vi "VI Tree.vi"   [LabVIEW 2016, in "Error Manager.lvlib"]
doc: "VI Tree\nThis VI lists all the public VIs and CTLs of the library."
uses:
  Error Manager.lvlib
  Show Error Window Instruction (enum).ctl
panel:
  # "VI Tree\nSee the block diagram for the VI Tree"
types:
  T1 = typedef "Error Manager.lvlib/Show Error Window Instruction (enum).ctl" = enum16{"Use Default Setting", "Show", "Do Not Show"}
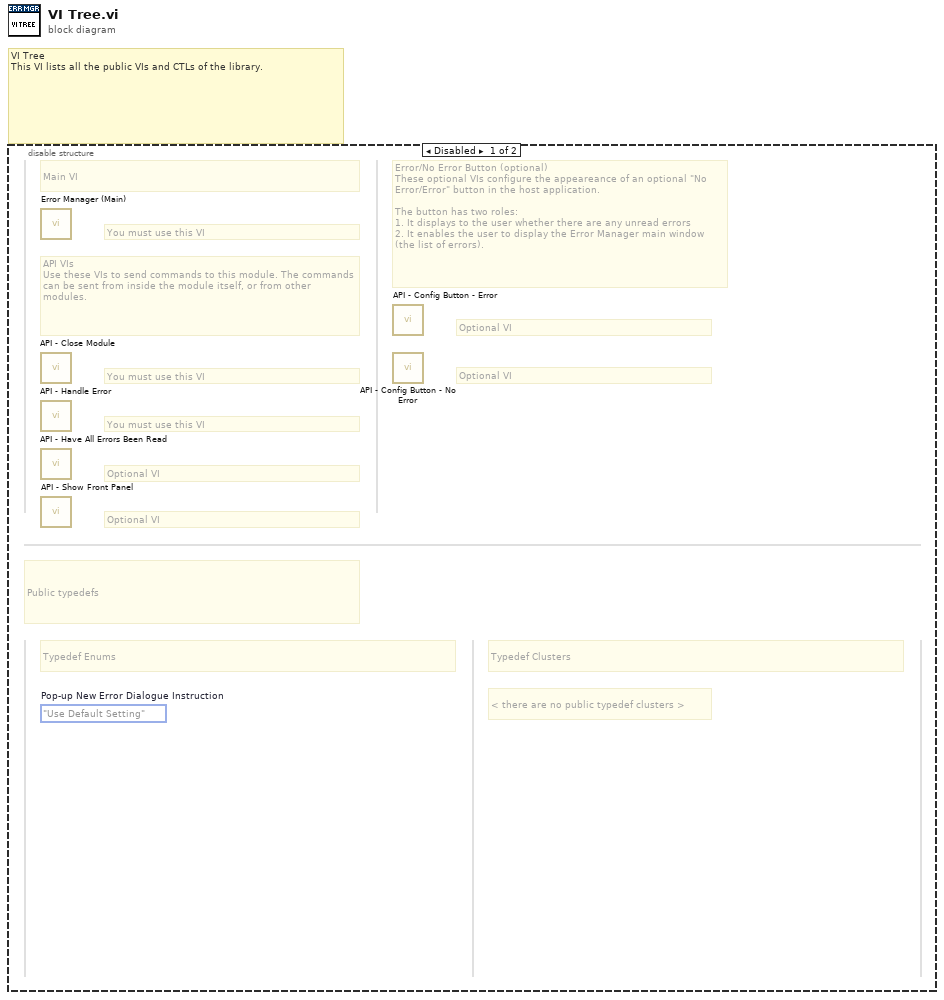
[diagram p0: block diagram]
diagram:
  # "VI Tree\nThis VI lists all the public VIs and CTLs of the library."
  n1 = disable-structure shown="Disabled" {
    frame Disabled {
      (unwired) Show_Error_Window_Instruction_(enum)."Use Default Setting"  # Pop-up New Error Dialogue Instruction
      # "Optional VI"
      # "Optional VI"
      # "Optional VI"
      # "Optional VI"
      # "You must use this VI"
      # "You must use this VI"
      # "You must use this VI"
      # "Error/No Error Button (optional)\nThese optional VIs configure the appeareance of an optional \"No Error/Error\" button in the host application.\n\nThe button has two roles:\n1. It displays to the user whether there are any unread errors\n2. It enables the user to display the Error Manager main window (the list of errors)."
      # "API VIs\nUse these VIs to send commands to this module. The commands can be sent from inside the module itself, or from other modules."
      # "Main VI"
      # "< there are no public typedef clusters >"
      # "Typedef Clusters"
      # "Typedef Enums"
      # "Public typedefs"
      n2 = call "Error Manager (Main).vi"() -> ()  [unwired: 11 in, 1 out]
      n3 = call "API - Close Module.vi"() -> ()  [unwired: 11 in, 1 out]
      n4 = call "API - Handle Error.vi"() -> ()  [unwired: 11 in, 1 out]
      n5 = call "API - Have All Errors Been Read.vi"() -> ()  [unwired: 10 in, 2 out]
      n6 = call "API - Show Front Panel.vi"() -> ()  [unwired: 11 in, 1 out]
      n7 = call "API - Config Button - Error.vi"() -> ()  [unwired: 11 in, 1 out]
      n8 = call "API - Config Button - No Error.vi"() -> ()  [unwired: 11 in, 1 out]
    }
    frame Enabled {
    }
  }
